vi "Test4.vi"() -> ()   [LabVIEW 2013]
panel:
  out "standard error":string
  out "standard output":string
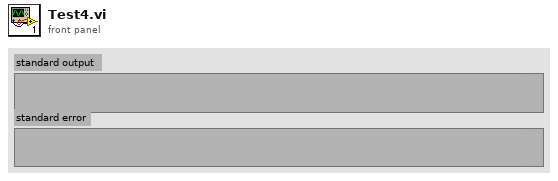
[diagram p1: front panel]
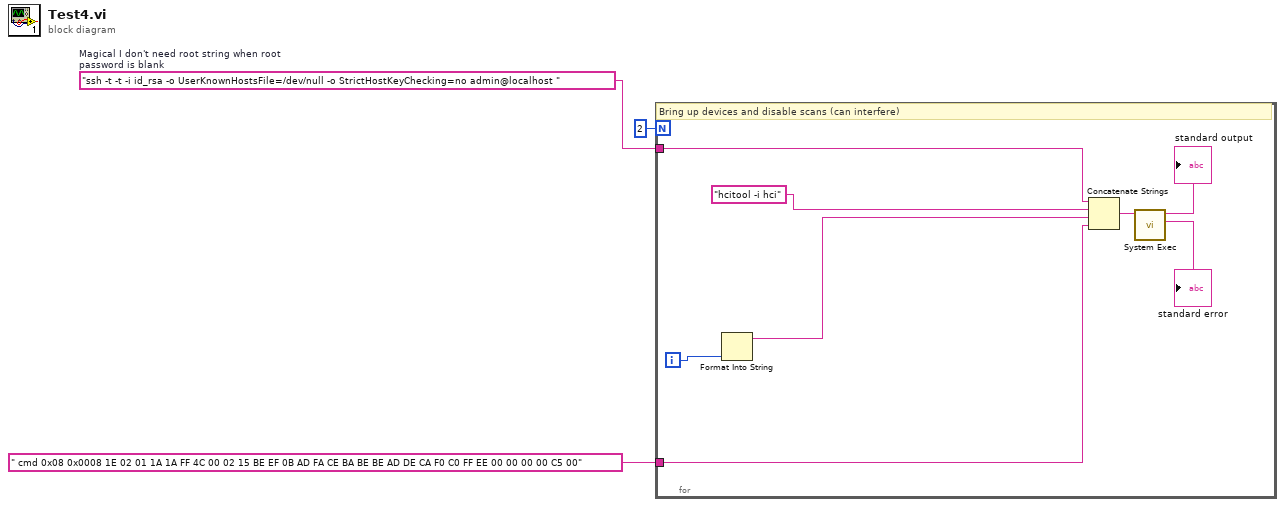
[diagram p0: block diagram]
diagram:
  w3 = "ssh -t -t -i id_rsa -o UserKnownHostsFile=/dev/null -o StrictHostKeyChecking=no admin@localhost "  # Magical I don't need root string when root password is blank
  n1 = for {
    N: 2 -> [_]
    tunnel: w3 -> [w9]
    tunnel: " cmd 0x08 0x0008 1E 02 01 1A 1A FF 4C 00 02 15 BE EF 0B AD FA CE BA BE BE AD DE CA F0 C0 FF EE 00 00 00 00 C5 00" ("command line") -> [w4]
    i -> [w11]
    # "Bring up devices and disable scans (can interfere)"
    n2 = Format Into String(w11) -> (resulting string=w5:string)  [unwired: 3 in, 1 out]
    n3 = Concatenate Strings(w9, "hcitool -i hci", w5, w4) -> (w10:string)
    n4 = call <vilib>:"System Exec.vi"("command line"=w10) -> ("standard error"=→"standard error":string, "standard output"=→"standard output":string)  [unwired: 7 in, 2 out]
  }
